vi "Change Active Instrument.vi"(8 "error in":errorcluster, 9 "Panel":i32, 10 "Identifier":string, 11 "Manual UI in":refnum<class "Manual UI.lvclass">) -> (0 "error out":errorcluster, 3 "Manual UI out":refnum<class "Manual UI.lvclass">)   [LabVIEW 2019, in "Manual UI.lvlib" / "Manual UI.lvclass"]
uses:
  Project/Manual UI.lvclass
  builds/Engine/Panel Manager.lvlibp/Panel Actor Messages/Show Panel Msg/Show Panel Msg.lvclass
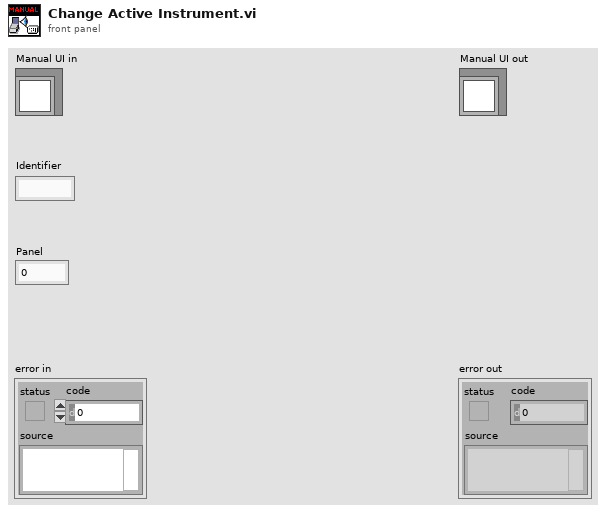
[diagram p1: front panel]
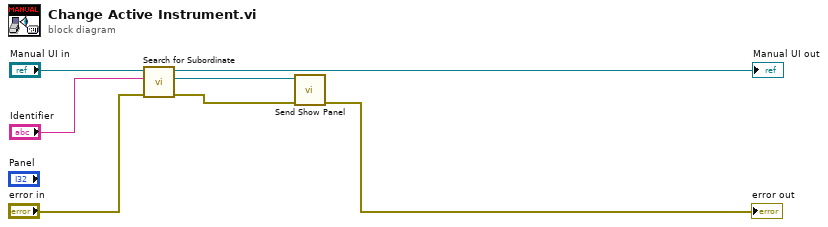
[diagram p0: block diagram]
diagram:
  n1 = call "Search for Subordinate.vi"("error in"="error in", "Identifier"="Identifier", "Manual UI in"="Manual UI in") -> ("error out"=w4:errorcluster, "Enqueuer"=w5:refnum<class "Message Enqueuer.lvclass">, "Manual UI out"=→"Manual UI out":refnum<class "Manual UI.lvclass">)  [unwired: 4 in, 2 out]
  n2 = call "Send Show Panel.vi"("Error In"=w4, "Message Enqueuer in"=w5) -> ("Error Out"=→"error out":errorcluster)  [unwired: 8 in, 1 out]
